vi "Configure Acquisition Trigger Source.vi"(8 "error in (no error)":errorcluster, 10 "Acquisition Trigger Source (0: Bus)":u16(ring) items=["Bus", "Voltage Trigger", "Current Trigger", "External", "Pin 1 ", "Pin 2", "Pin 3", "Pin 4", "Pin 5", "Pin 6", "Pin 7", "Transient"], 11 "VISA resource name":refnum<visa-resource-name>) -> (0 "error out":errorcluster, 3 "VISA resource name out":refnum<visa-resource-name>)   [LabVIEW 2019, in "Agilent N7976A.lvlib"]
doc: "Selects the trigger source for the acquisition system."
uses:
  <instrlib>/Agilent N7976A/Agilent N7976A.lvlib
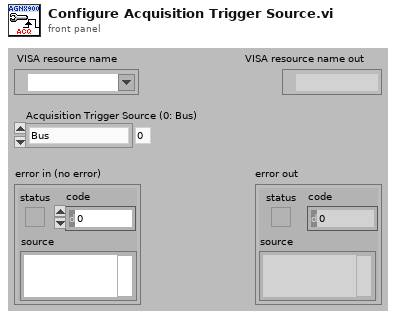
[diagram p1: front panel]
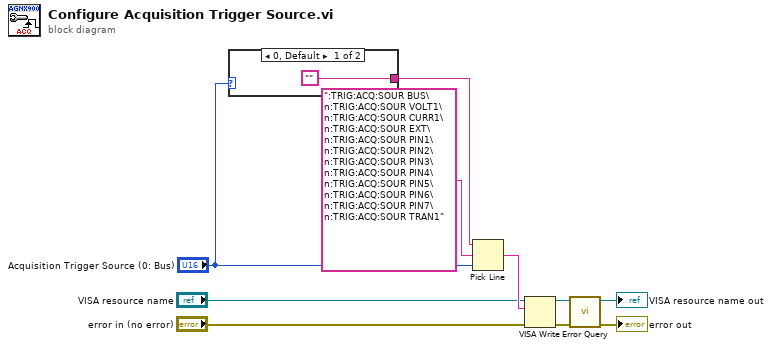
[diagram p0: block diagram]
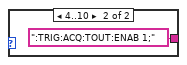
[diagram p2: hidden frame]
diagram:
  n1 = case shown="0, Default" "Acquisition Trigger Source (0: Bus)" {
    tunnel: ["" ("string (\"\")") ":TRIG:ACQ:TOUT:ENAB 1;" ("string (\"\")")] -> w2
    frame 0, Default {
    }
    frame 4..10 {
    }
  }
  n2 = Pick Line(string ("")=w2, multi-line string=":TRIG:ACQ:SOUR BUS\n:TRIG:ACQ:SOUR VOLT1\n:TRIG:ACQ:SOUR CURR1\n:TRIG:ACQ:SOUR EXT\n:TRIG:ACQ:SOUR PIN1\n:TRIG:ACQ:SOUR PIN2\n:TRIG:ACQ:SOUR PIN3\n:TRIG:ACQ:SOUR PIN4\n:TRIG:ACQ:SOUR PIN5\n:TRIG:ACQ:SOUR PIN6\n:TRIG:ACQ:SOUR PIN7\n:TRIG:ACQ:SOUR TRAN1", line index="Acquisition Trigger Source (0: Bus)") -> (output string=w8:string)
  n3 = VISA Write(VISA resource name="VISA resource name", write buffer=w8, error in (no error)="error in (no error)") -> (VISA resource name out=w9:refnum<visa-resource-name>, error out=w10:errorcluster)  [unwired: 1 out]
  n4 = call <instrlib>:"Error Query.vi"("error in (no error)"=w10, "VISA resource name"=w9) -> ("error out"=→"error out":errorcluster, "VISA resource name out"=→"VISA resource name out":refnum<visa-resource-name>)  [unwired: 6 in, 2 out]
